vi "CommonVIs_ConvertStringToHex.vi"(2 "inputString":string, 5 "error in (no error)":errorcluster) -> (16 "outputString":string, 19 "error out":errorcluster)   [LabVIEW 2012]
doc: "Convert a string to an array of hex data. Used to compare to strings"
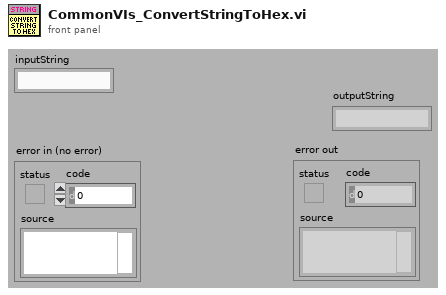
[diagram p1: front panel]
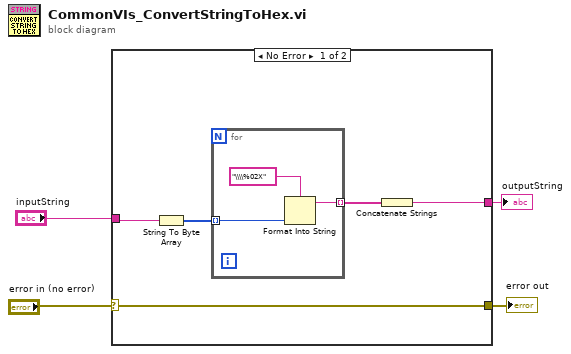
[diagram p0: block diagram]
diagram:
  n1 = case shown="No Error" "error in (no error)" {
    selector: "error in (no error)" -> [w5 w14]
    tunnel: [w5 w14] -> w3
    tunnel: "inputString" -> [w9 _]
    tunnel: [w6 "ERROR"] -> w1
    frame No Error {
      n2 = String To Byte Array(string=w9) -> (unsigned byte array=w8:u8[])
      n3 = for {
        tunnel: w8 -> [w12] mode=indexing
        tunnel: [w11] -> w7 mode=indexing
        n4 = Format Into String(format string="\\\\%02X" ("Input String"), w12) -> (resulting string=w11:string)  [unwired: 2 in, 1 out]
      }
      n5 = Concatenate Strings(w7) -> (w6:string)
    }
    frame Error {
      # "Error"
    }
  }
  "error out" <- w3
  "outputString" <- w1
